vi "binary record ch1.vi"(3 "xIncrement":dbl, 4 "Record":bool, 5 "gain":dbl=1.0, 6 "offset":dbl, 7 "relativeInitialX":dbl, 8 "Index files\npath array":i32, 9 "Files path array":path[](array[path]), 10 "wfm":i16[][](array[numeric]), 11 "reference":refnum<vi>) -> ()   [LabVIEW 2011]
panel:
  out "error out":errorcluster
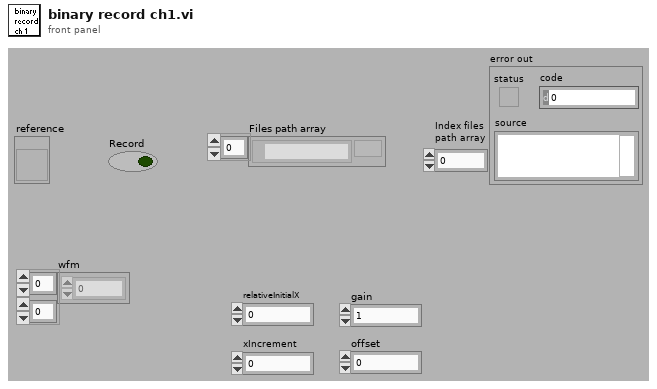
[diagram p1: front panel]
types:
  T1 = enum16{"open", "replace", "create", "open or create", "replace or create", "replace or create with confirmation"}
  T2 = enum16{"big-endian, network order", "native, host order", "little-endian"}
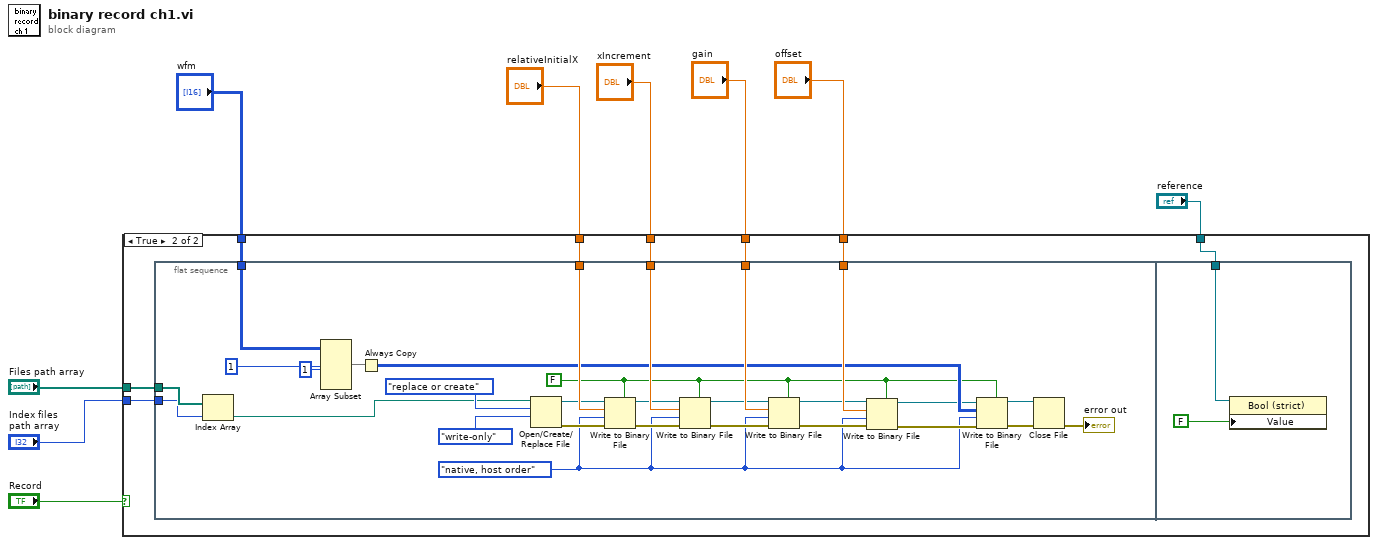
[diagram p0: block diagram]
diagram:
  n1 = case shown="True" "Record" {
    tunnel: "wfm" -> [_ w17]
    tunnel: "relativeInitialX" -> [_ w16]
    tunnel: "xIncrement" -> [_ w15]
    tunnel: "gain" -> [_ w14]
    tunnel: "offset" -> [_ w13]
    tunnel: "reference" -> [_ w12]
    tunnel: "Files path array" -> [_ w11]
    tunnel: "Index files\npath array" -> [_ w10]
    frame False {
    }
    frame True {
      n2 = flat-sequence {
        tunnel: w17 -> [w46]
        tunnel: w16 -> [w45]
        tunnel: w15 -> [w44]
        tunnel: w14 -> [w43]
        tunnel: w13 -> [w42]
        tunnel: w11 -> [w22]
        tunnel: w10 -> [w20]
        tunnel: w12 -> [w47]
        frame #0 {
          w24 = FALSE ("prepend array or string size? (T)")
          w25 = T2."native, host order" ("byte order (0:big-endian, network order)")
          n3 = Index Array(array=w22, index=w20) -> (element=w23:path)
          n4 = Array Subset(array=w46, index (row)=1 ("index"), length (row)=1 ("length")) -> (w38:i16[][])  [unwired: 2 in]
          n5 = Always Copy(1:w38) -> (0:w39:i16[][])
          n6 = Open/Create/Replace File(file path (use dialog)=w23, operation (0:open)=T1."replace or create", access (0:read/write)=enum16{"read/write", "read-only", "write-only"}."write-only") -> (refnum out=w37:refnum<file>, error out=w36:errorcluster)  [unwired: 1 in, 3 out]
          n7 = Write to Binary File(file (use dialog)=w37, data=w45, error in=w36, 5:w24, 9:w25) -> (refnum out=w35:refnum<file>, error out=w34:errorcluster)  [unwired: 2 out]
          n8 = Write to Binary File(file (use dialog)=w35, data=w44, error in=w34, 5:w24, 9:w25) -> (refnum out=w33:refnum<file>, error out=w29:errorcluster)  [unwired: 2 out]
          n9 = Write to Binary File(file (use dialog)=w33, data=w43, error in=w29, 5:w24, 9:w25) -> (refnum out=w32:refnum<file>, error out=w28:errorcluster)  [unwired: 2 out]
          n10 = Write to Binary File(file (use dialog)=w32, data=w42, error in=w28, 5:w24, 9:w25) -> (refnum out=w31:refnum<file>, error out=w27:errorcluster)  [unwired: 2 out]
          n11 = Write to Binary File(file (use dialog)=w31, data=w39, error in=w27, 5:w24, 9:w25) -> (refnum out=w30:refnum<file>, error out=w26:errorcluster)  [unwired: 2 out]
          n12 = Close File(refnum=w30, error in=w26) -> (error out=→"error out":errorcluster)  [unwired: 1 out]
        }
        frame #1 {
          n13 = property on="Property Node" class="Bool (strict)"(reference=w47, "Value"=FALSE ("Boolean")) -> ()  [unwired: 1 in, 2 out]
        }
      }
    }
  }
